vi "WaveformSplit.vi"(3 "signal in":waveform(dbl) caption="Waveform In", 7 "Duration":dbl, 9 "error in (no error)":errorcluster) -> (0 "A":waveform(dbl) caption="Waveform 1", 1 "B":waveform(dbl) caption="Waveform 2", 6 "error out":errorcluster)   [LabVIEW 2009]
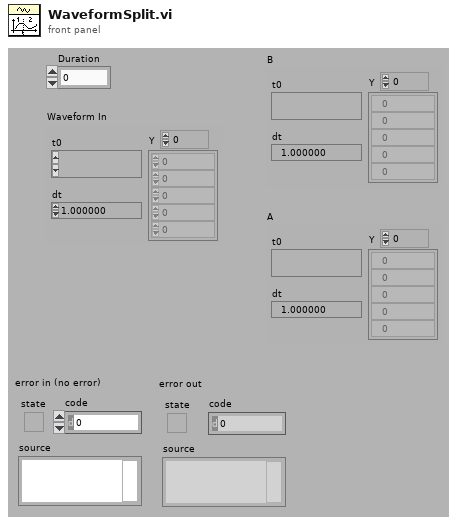
[diagram p1: front panel]
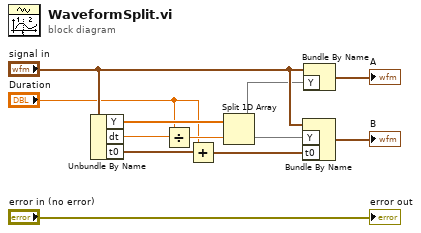
[diagram p0: block diagram]
diagram:
  n1 = Unbundle By Name("signal in") -> ("Y"=w9:dbl[], "dt"=w3:dbl, "t0"=w2:timestamp)
  n2 = Divide(x="Duration", y=w3) -> (x/y=w8:dbl)
  n3 = Add(x=w2, y="Duration") -> (x+y=w5:timestamp)
  n4 = Split 1D Array(array=w9, index=w8) -> (first subarray=w7:dbl[], second subarray=w6:dbl[])
  n5 = Bundle By Name(cluster="signal in", "Y"=w6, "t0"=w5) -> (→"B":waveform(dbl))
  n6 = Bundle By Name(cluster="signal in", "Y"=w7) -> (→"A":waveform(dbl))
  "error out" <- "error in (no error)"
